vi "T_Sat_Curve_Fit_R134a.vi"(8 "error in (no error)":errorcluster, 11 "Waveform in":waveform(dbl)) -> (0 "error out":errorcluster, 3 "Waveform out":waveform(dbl))   [LabVIEW 2016]
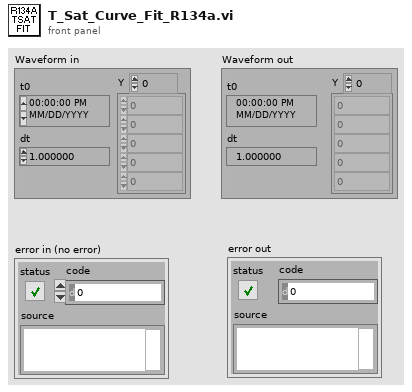
[diagram p1: front panel]
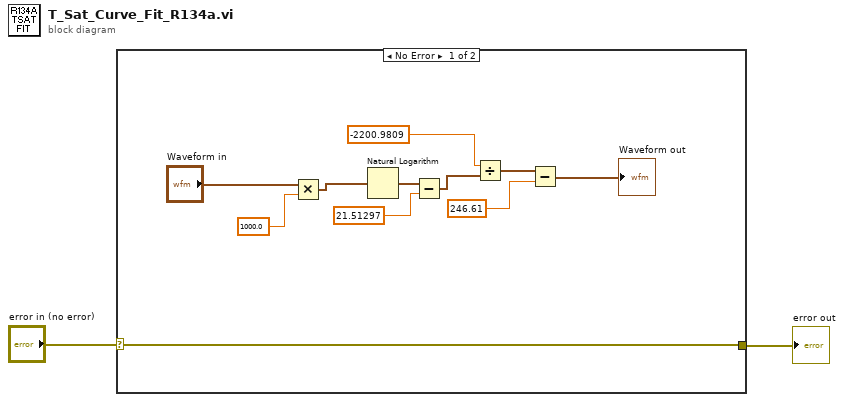
[diagram p0: block diagram]
diagram:
  n1 = case shown="No Error" "error in (no error)" {
    selector: "error in (no error)" -> [w3 w14]
    tunnel: [w3 w14] -> w1
    frame No Error {
      n2 = Multiply(x="Waveform in", y=1000.0) -> (x*y=w10:waveform(dbl))
      n3 = Natural Logarithm(1:w10) -> (0:w9:waveform(dbl))
      n4 = Subtract(x=w9, y=21.51297) -> (x-y=w6:waveform(dbl))
      n5 = Divide(x=-2200.9809, y=w6) -> (x/y=w5:waveform(dbl))
      n6 = Subtract(x=w5, y=246.61) -> (x-y=→"Waveform out":waveform(dbl))
    }
    frame Error {
    }
  }
  "error out" <- w1
